vi "Error Template.vi"   [LabVIEW 2016]
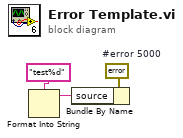
[diagram p0: block diagram]
diagram:
  w1 = errorcluster {"status"=TRUE, "code"=533, "source"="test%d"}  # #error 5000
  n1 = Format Into String(format string="test%d") -> (resulting string=w2:string)  [unwired: 3 in, 1 out]
  n2 = Bundle By Name(cluster=w1, "source"=w2) -> ()  [unwired: 1 out]
